vi "HEX to I32 NEW.vi"(10 "Numeric":i32, 11 "字符串":string="\u0000\u0000œ@") -> (3 "(hi.lo)":i32)   [LabVIEW 2017]
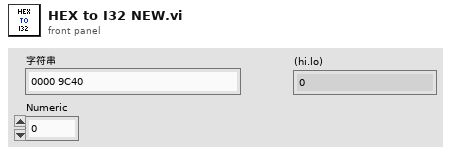
[diagram p1: front panel]
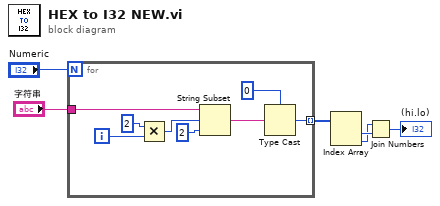
[diagram p0: block diagram]
diagram:
  n1 = for {
    N: "Numeric" -> [_]
    tunnel: "字符串" -> [w14]
    tunnel: [w7] -> w4 mode=indexing
    i -> [w10]
    n2 = Multiply(x=2, y=w10) -> (x*y=w11:i32)
    n3 = String Subset(string=w14, offset (0)=w11, length (rest)=2 ("length (rest)")) -> (substring=w9:string)
    n4 = Type Cast(type=i16 0 ("lo(x) 2"), x=w9) -> (*(type *) &x=w7:i16)
  }
  n5 = Index Array(array=w4) -> (element #1=w3:i16, element #2=w2:i16)  [unwired: 2 in]
  n6 = Join Numbers(hi=w2, lo=w3) -> ((hi.lo)=→"(hi.lo)":u32)
